vi "VL53L0X_ValidateI2C.vi"(11 "REV2mDistanceSensorDevRef":T1) -> (3 "REV2mDistanceSensorDevRef Out":T1)   [LabVIEW 2019, in "DistanceSensorDriver.lvlib"]
uses:
  DistanceSensorDriver.lvlib
  Typedef/REV2mDistanceSensorDevRef.ctl
  Typedef/Ports.ctl
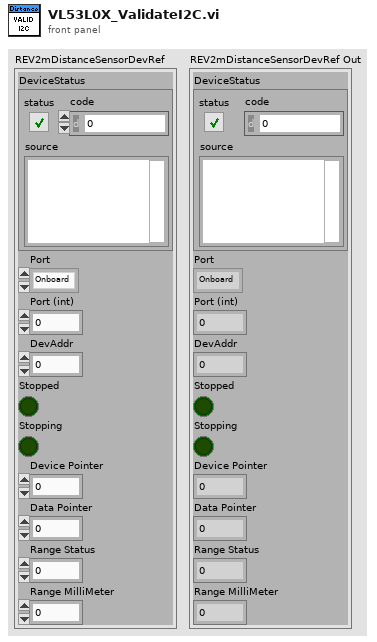
[diagram p1: front panel]
types:
  T1 = typedef "DistanceSensorDriver.lvlib/REV2mDistanceSensorDevRef.ctl" = cluster{"DeviceStatus":errorcluster, "Port":T2, "Port (int)":i32, "DevAddr":i32, "Stopped":bool, "Stopping":bool, "Device Pointer":u64, "Data Pointer":u64, "Range Status":u8, "Range MilliMeter":u16}
  T2 = typedef "DistanceSensorDriver.lvlib/Ports.ctl" = enum32{"Onboard", "MXP"}
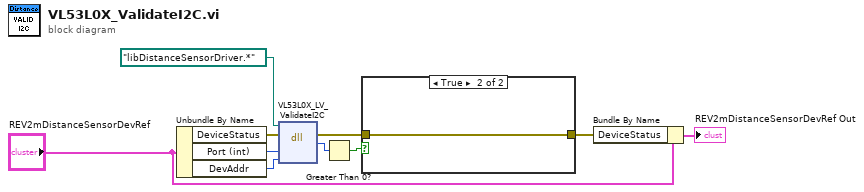
[diagram p0: block diagram]
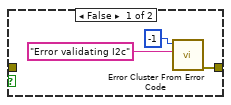
[diagram p2: hidden frame]
diagram:
  n1 = Unbundle By Name("REV2mDistanceSensorDevRef") -> ("DeviceStatus"=w6:errorcluster, "Port (int)"=w5:i32, "DevAddr"=w4:i32)
  n2 = dll-call lib="?" fn="VL53L0X_LV_ValidateI2C"(path in=path "libDistanceSensorDriver.*", error in=w6, "port"=w5, "addr"=w4) -> (error out=w7:errorcluster, "return type"=w9:i32)  [unwired: 3 in, 1 out]
  n3 = Greater Than 0?(x=w9) -> (x > 0?=w8:bool)
  n4 = case shown="True" w8 {
    tunnel: [w11 w14] -> w3
    tunnel: w7 -> [_ w14]
    frame False {
      n5 = call <vilib>:"Error Cluster From Error Code.vi"("error message (\"\")"="Error validating I2c" ("error message (\"\")"), "error code (0)"=-1) -> ("error out"=w11:errorcluster)  [unwired: 7 in]
    }
    frame True {
    }
  }
  n6 = Bundle By Name(cluster="REV2mDistanceSensorDevRef", "DeviceStatus"=w3) -> (→"REV2mDistanceSensorDevRef Out":T1)
